vi "Create.vi"(8 "error in (no error)":errorcluster) -> (0 "error out":errorcluster, 3 "View out":refnum<class "View.lvclass">)   [LabVIEW 2020, in "View.lvclass"]
uses:
  View.lvclass
  View.lvclass/View.ctl
  Controller/Controller.lvclass
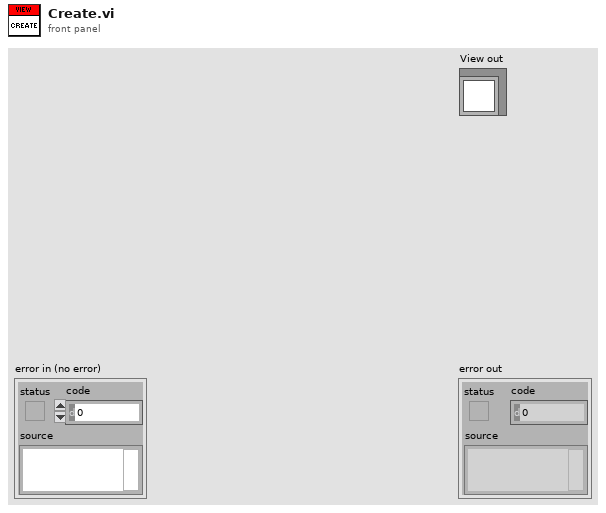
[diagram p1: front panel]
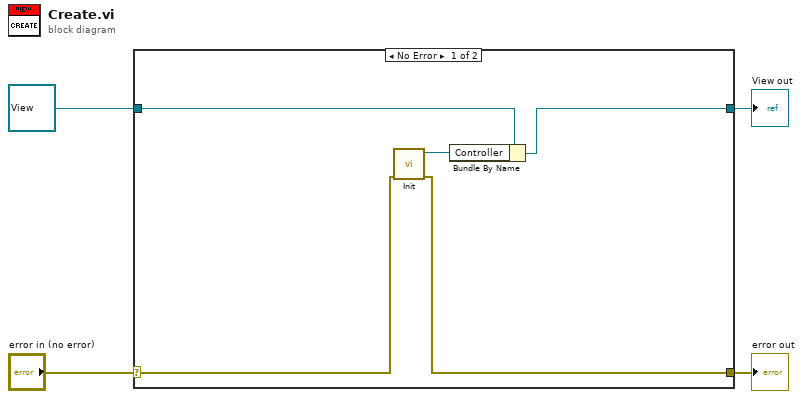
[diagram p0: block diagram]
diagram:
  n1 = case shown="No Error" "error in (no error)" {
    selector: "error in (no error)" -> [w7 w11]
    tunnel: [w6 w11] -> w3
    tunnel: [w5 w10] -> w2
    tunnel: refnum<class "View.lvclass"> refnum ("View in") -> [w9 w10]
    frame No Error {
      n2 = call "Init.vi"("error in (no error)"=w7) -> ("error out"=w6:errorcluster, "Controller out"=w8:refnum<class "Controller.lvclass">)  [unwired: 9 in]
      n3 = Bundle By Name(cluster=w9, "Controller"=w8) -> (w5:refnum<class "View.lvclass">)
    }
    frame Error {
    }
  }
  "error out" <- w3
  "View out" <- w2
